vi "Generate Error if Invalid.vi"(7 "chain levels to remove (2)":i32=2 min=1, 8 "error in (no error)":errorcluster, 11 "starter kit host in":refnum<class "NI_Robotics_Starter Kit Host.lvclass">) -> (0 "error out":errorcluster, 2 "valid?":bool, 3 "starter kit host out":refnum<class "NI_Robotics_Starter Kit Host.lvclass">)   [LabVIEW 2017, in "NI_Robotics_Starter Kit Host.lvclass"]
uses:
  <vilib>/robotics/Starter Kit/Host Interface/NI_Robotics_Starter Kit Host.lvclass
  <vilib>/robotics/Utilities/NI_Robotics Utilities.lvlib
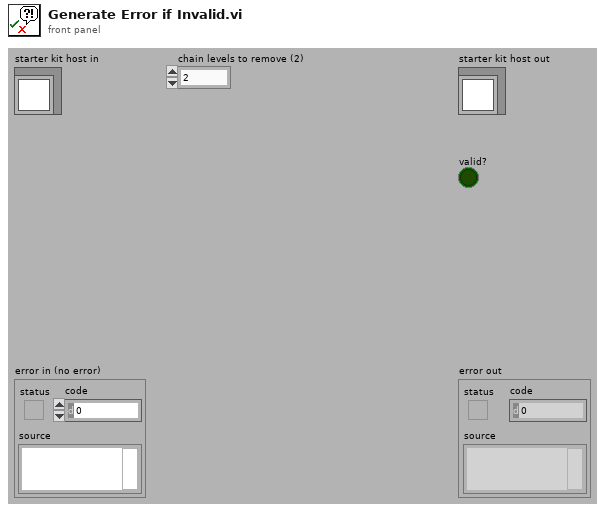
[diagram p1: front panel]
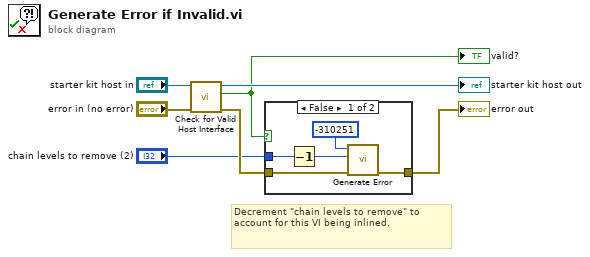
[diagram p0: block diagram]
diagram:
  # "Decrement \"chain levels to remove\" to account for this VI being inlined."
  n1 = call-dynamic "Check for Valid Host Interface.vi"("error in (no error)"="error in (no error)", "starter kit host in"="starter kit host in") -> ("error out"=w2:errorcluster, "valid?"=w3:bool, "starter kit host out"=→"starter kit host out":refnum<class "NI_Robotics_Starter Kit Host.lvclass">)  [unwired: 7 in]
  "valid?" <- w3
  n2 = case shown="False" w3 {
    tunnel: w2 -> [w11 w13]
    tunnel: [w10 w13] -> w6
    tunnel: "chain levels to remove (2)" -> [w9 _]
    frame False {
      n3 = Decrement(x=w9) -> (x-1=w8:i32)
      n4 = call <vilib>:"Generate Error.vi"("error in (no error)"=w11, "chain levels to remove (1)"=w8, "code"=-310251) -> ("error out"=w10:errorcluster)  [unwired: 8 in]
    }
    frame True {
    }
  }
  "error out" <- w6
